vi "GUI_Final.vi"() -> ()   [LabVIEW 2013]
uses:
  <vilib>/Instr/_visa.llb/VISA Configure Serial Port (Instr).vi
panel:
  out "Angle":u8[](array[numeric])
  out "Left":bool
  out "Right":bool
  out "read buffer":string
  in  "Stop":bool
  in  "Angle":string
  out "Error":errorcluster
  out "Arduino Data":string
  in  "Mode":bool
  in  "Baud Rate 2":u32=9600
  in  "Port 2":refnum<visa-resource-name>
  in  "Baud Rate":u32=9600
  in  "Port":refnum<visa-resource-name>
  out "Response 2":string
  in  "Command":string
  out "error out":errorcluster
  out "Numeric 12":i32
  in  "angle":i32
  in  "OK":bool
  in  "Commands":string(combo)
  out "error out 2":errorcluster
  in  "MODE":bool
  # "Arduino Interface"
  # "Encoder Interface"
  # "Text Mode"
  # "Button Mode"
  # "Select : ON : Text Mode , \n              OFF : ButtonMode"
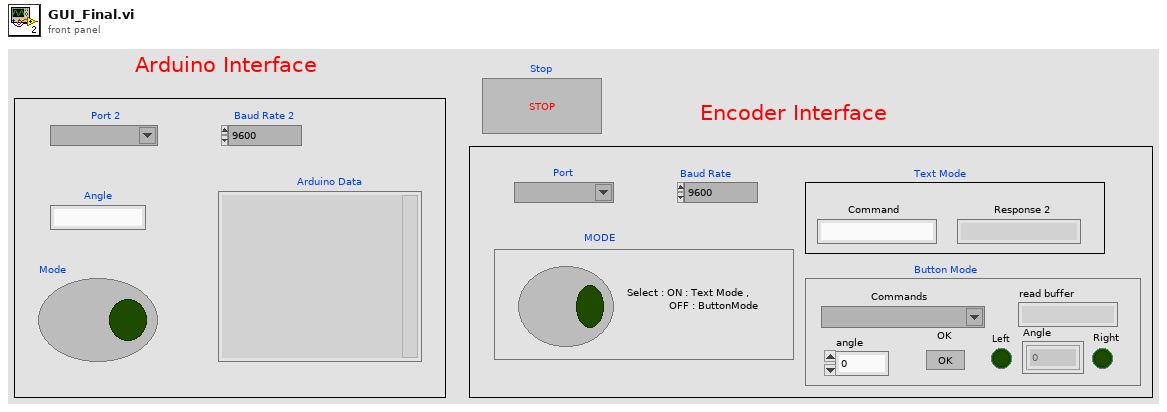
[diagram p1: front panel]
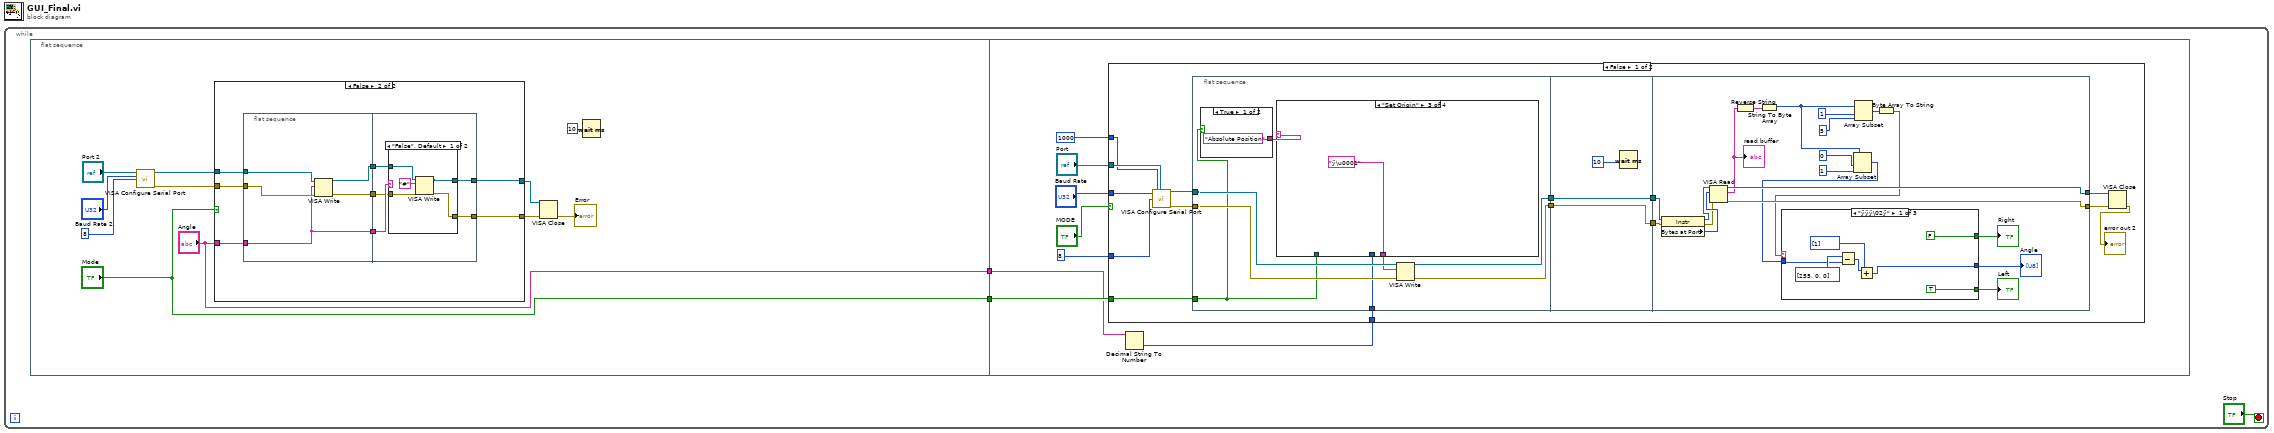
[diagram p0: block diagram]
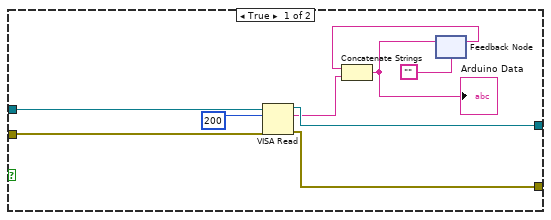
[diagram p2: hidden frame]
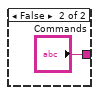
[diagram p4: hidden frame]
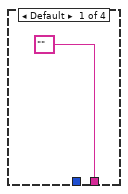
[diagram p5: hidden frame]
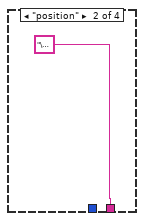
[diagram p6: hidden frame]
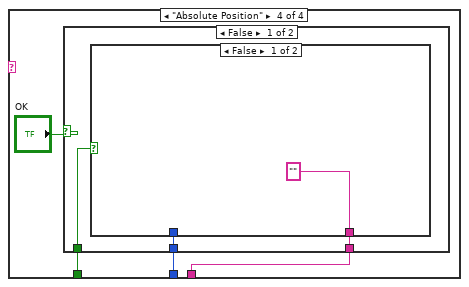
[diagram p7: hidden frame]
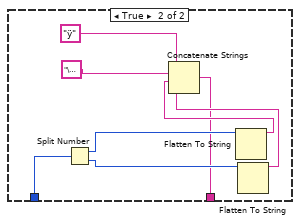
[diagram p8: hidden frame]
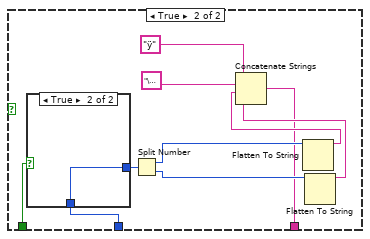
[diagram p9: hidden frame]
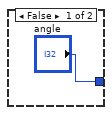
[diagram p10: hidden frame]
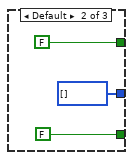
[diagram p11: hidden frame]
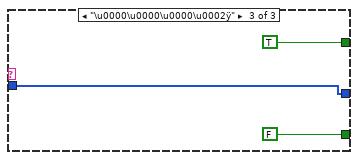
[diagram p12: hidden frame]
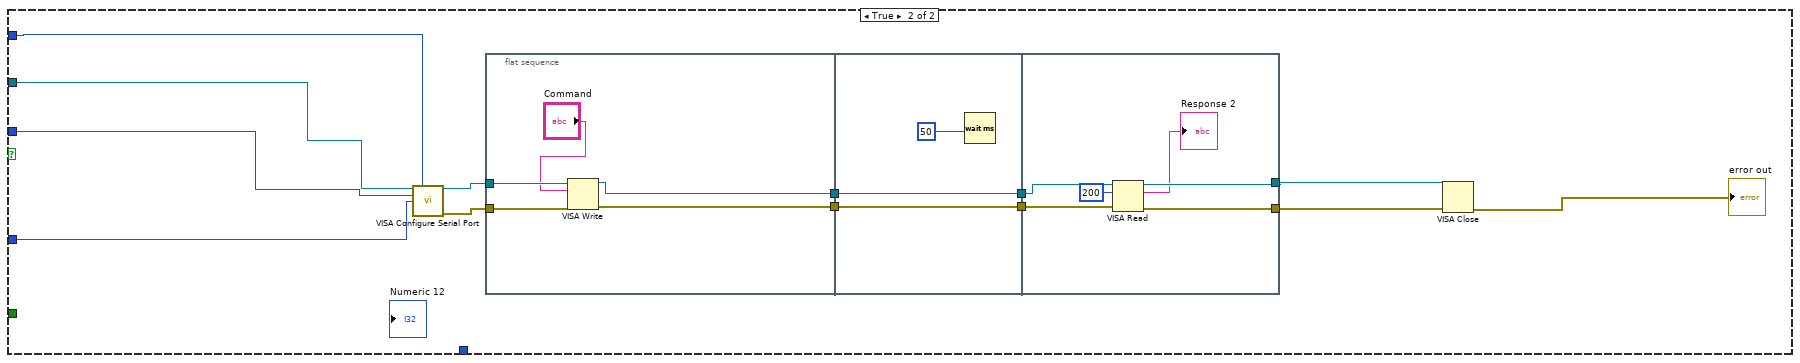
[diagram p13: hidden frame]
diagram:
  n1 = while {
    stop <- "Stop" stop-if-true
    n2 = flat-sequence {
      tunnel: ["Mode"] -> w3
      tunnel: ["Angle"] -> w2
      tunnel: w3 -> [w52]
      tunnel: w2 -> [w51]
      frame #0 {
        n3 = call-poly "VISA Configure Serial Port"("VISA resource name"="Port 2", "baud rate (9600)"="Baud Rate 2", "data bits (8)"=u16 8) -> ("VISA resource name out"=w6:refnum<visa-resource-name>, "error out"=w7:errorcluster)  [unwired: 11 in]
        n4 = case shown="False" "Mode" {
          tunnel: w6 -> [w21 w31]
          tunnel: [w22 w25] -> w13
          tunnel: [w23 w26] -> w14
          tunnel: w7 -> [w20 w30]
          tunnel: "Angle" -> [_ w24]
          frame True {
            n5 = VISA Read(VISA resource name=w21, byte count=u32 200, error in (no error)=w20) -> (VISA resource name out=w23:refnum<visa-resource-name>, read buffer=w18:string, error out=w22:errorcluster)  [unwired: 1 out]
            n6 = feedback #1("") -> (w17:string)
            n7 = Concatenate Strings(w17, w18) -> (w16:string)
            "Arduino Data" <- w16
            n8 = feedback-in #1(w16) -> ()
          }
          frame False {
            n9 = flat-sequence {
              tunnel: w31 -> [w36]
              tunnel: w30 -> [w35]
              tunnel: [w32] -> w29
              tunnel: [w34] -> w28
              tunnel: [w33] -> w27
              tunnel: w24 -> [w32]
              tunnel: w29 -> [w41]
              tunnel: w28 -> [w40]
              tunnel: w27 -> [w39]
              tunnel: [w38] -> w26
              tunnel: [w37] -> w25
              frame #0 {
                n10 = VISA Write(VISA resource name=w36, write buffer=w32, error in (no error)=w35) -> (VISA resource name out=w34:refnum<visa-resource-name>, error out=w33:errorcluster)  [unwired: 1 out]
              }
              frame #1 {
                n11 = case shown="\"False\", Default" w41 {
                  tunnel: w40 -> [w45 w48]
                  tunnel: w39 -> [w44 w47]
                  tunnel: [w43 w48] -> w38
                  tunnel: [w42 w47] -> w37
                  frame "False", Default {
                    n12 = VISA Write(VISA resource name=w45, write buffer="#", error in (no error)=w44) -> (VISA resource name out=w43:refnum<visa-resource-name>, error out=w42:errorcluster)  [unwired: 1 out]
                  }
                  frame "" {
                  }
                }
              }
            }
          }
        }
        n13 = VISA Close(VISA resource name=w14, error in (no error)=w13) -> (error out=→"Error":errorcluster)
        n14 = Wait (ms)(milliseconds to wait=u32 10) -> ()  [unwired: 1 out]
      }
      frame #1 {
        n15 = Decimal String To Number(string=w51) -> (number=w49:i32)  [unwired: 2 in, 1 out]
        n16 = case shown="False" "MODE" {
          tunnel: u32 1000 ("timeout (10sec)") -> [w57 w152]
          tunnel: "Port" -> [w65 w151]
          tunnel: "Baud Rate" -> [w64 w150]
          tunnel: u16 8 ("data bits (8)") -> [w59 w149]
          tunnel: w52 -> [w63 _]
          tunnel: w49 -> [w58 _]
          frame False {
            n17 = call-poly "VISA Configure Serial Port"("VISA resource name"=w65, "timeout (10sec)"=w57, "baud rate (9600)"=w64, "data bits (8)"=w59) -> ("VISA resource name out"=w69:refnum<visa-resource-name>, "error out"=w68:errorcluster)  [unwired: 10 in]
            n18 = flat-sequence {
              tunnel: [w78] -> w71
              tunnel: w69 -> [w77]
              tunnel: w68 -> [w76]
              tunnel: [w79] -> w67
              tunnel: w63 -> [w73]
              tunnel: w58 -> [w72]
              tunnel: [w114] -> w70
              tunnel: w71 -> [w113]
              tunnel: w67 -> [w114]
              tunnel: [w113] -> w66
              tunnel: w70 -> [w121]
              tunnel: [w135] -> w61
              tunnel: [w134] -> w62
              tunnel: w66 -> [w132]
              frame #0 {
                n19 = case shown="True" w73 {
                  tunnel: ["Absolute Position" ("Commands") "Commands"] -> w75
                  frame True {
                  }
                  frame False {
                  }
                }
                n20 = case shown="\"Set Origin\"" w75 {
                  tunnel: ["" "\u001f" "ÿ\u0001" w85] -> w74
                  tunnel: w73 -> [_ _ _ w87]
                  tunnel: w72 -> [_ _ _ w86]
                  frame Default {
                  }
                  frame "position" {
                  }
                  frame "Set Origin" {
                  }
                  frame "Absolute Position" {
                    n21 = case shown="False" "OK" {
                      tunnel: w87 -> [w91 w103]
                      tunnel: w86 -> [w90 w101]
                      tunnel: [w89 w102] -> w85
                      frame False {
                        n22 = case shown="False" w91 {
                          tunnel: w90 -> [_ w94]
                          tunnel: ["" w93] -> w89
                          frame False {
                          }
                          frame True {
                            n23 = Split Number(x=w94) -> (hi(x)=w96:u16, lo(x)=w95:u16)
                            n24 = Flatten To String(anything=w96) -> (data string=w98:string)  [unwired: 3 in, 2 out]
                            n25 = Flatten To String(anything=w95) -> (data string=w97:string)  [unwired: 3 in, 2 out]
                            n26 = Concatenate Strings("ÿ" ("string"), "\u0002" ("string"), w98, w97) -> (w93:string)
                          }
                        }
                      }
                      frame True {
                        n27 = case shown="True" w103 {
                          tunnel: w101 -> [_ w112]
                          tunnel: ["angle" w112] -> w104
                          frame False {
                          }
                          frame True {
                          }
                        }
                        n28 = Split Number(x=w104) -> (hi(x)=w106:u16, lo(x)=w105:u16)
                        n29 = Flatten To String(anything=w106) -> (data string=w108:string)  [unwired: 3 in, 2 out]
                        n30 = Flatten To String(anything=w105) -> (data string=w107:string)  [unwired: 3 in, 2 out]
                        n31 = Concatenate Strings("ÿ" ("string"), "\u0002" ("string"), w108, w107) -> (w102:string)
                      }
                    }
                  }
                }
                n32 = VISA Write(VISA resource name=w77, write buffer=w74, error in (no error)=w76) -> (VISA resource name out=w79:refnum<visa-resource-name>, error out=w78:errorcluster)  [unwired: 1 out]
              }
              frame #1 {
                n33 = Wait (ms)(milliseconds to wait=u32 10) -> ()  [unwired: 1 out]
              }
              frame #2 {
                n34 = property class="Instr"(reference=w121, error in=w132) -> (reference out=w120:refnum<visa-resource-name>, error out=w131:errorcluster, "Bytes at Port"=w133:u32)
                n35 = VISA Read(VISA resource name=w120, byte count=w133, error in (no error)=w131) -> (VISA resource name out=w134:refnum<visa-resource-name>, read buffer=w127:string, error out=w135:errorcluster)  [unwired: 1 out]
                "read buffer" <- w127
                n36 = Reverse String(1:w127) -> (0:w119:string)
                n37 = String To Byte Array(string=w119) -> (unsigned byte array=w130:u8[])
                n38 = Array Subset(array=w130, index=0, length=1) -> (w122:u8[])
                n39 = Array Subset(array=w130, index=1, length=5) -> (w123:u8[])
                n40 = Byte Array To String(unsigned byte array=w123) -> (string=w128:string)
                n41 = case shown="\"ÿÿÿ\\02ÿ\"" w128 {
                  tunnel: w122 -> [w139 _ w148]
                  tunnel: [w138 u8[] [] w148] -> w124
                  tunnel: [TRUE ("Boolean") FALSE ("Boolean") FALSE ("Boolean")] -> w126
                  tunnel: [FALSE ("Boolean") FALSE ("Boolean") TRUE ("Boolean")] -> w125
                  frame "ÿÿÿ\u0002ÿ" {
                    n42 = Subtract(x=u8[] [255, 0, 0] ("y"), y=w139) -> (x-y=w142:u8[])
                    n43 = Add(x=w142, y=u8[] [1]) -> (x+y=w138:u8[])
                  }
                  frame Default {
                  }
                  frame "\u0000\u0000\u0000\u0002ÿ" {
                  }
                }
                "Left" <- w126
                "Right" <- w125
                "Angle" <- w124
              }
            }
            n44 = VISA Close(VISA resource name=w62, error in (no error)=w61) -> (error out=→"error out 2":errorcluster)
          }
          frame True {
            n45 = call-poly "VISA Configure Serial Port"("VISA resource name"=w151, "timeout (10sec)"=w152, "baud rate (9600)"=w150, "data bits (8)"=w149) -> ("VISA resource name out"=w157:refnum<visa-resource-name>, "error out"=w156:errorcluster)  [unwired: 10 in]
            n46 = flat-sequence {
              tunnel: w157 -> [w164]
              tunnel: w156 -> [w166]
              tunnel: [w163] -> w161
              tunnel: [w165] -> w160
              tunnel: [w168] -> w159
              tunnel: w161 -> [w168]
              tunnel: [w167] -> w158
              tunnel: w160 -> [w167]
              tunnel: w159 -> [w175]
              tunnel: w158 -> [w174]
              tunnel: [w173] -> w154
              tunnel: [w172] -> w155
              frame #0 {
                n47 = VISA Write(VISA resource name=w164, write buffer="Command", error in (no error)=w166) -> (VISA resource name out=w163:refnum<visa-resource-name>, error out=w165:errorcluster)  [unwired: 1 out]
              }
              frame #1 {
                n48 = Wait (ms)(milliseconds to wait=u32 50) -> ()  [unwired: 1 out]
              }
              frame #2 {
                n49 = VISA Read(VISA resource name=w175, byte count=u32 200, error in (no error)=w174) -> (VISA resource name out=w172:refnum<visa-resource-name>, read buffer=→"Response 2":string, error out=w173:errorcluster)  [unwired: 1 out]
              }
            }
            n50 = VISA Close(VISA resource name=w155, error in (no error)=w154) -> (error out=→"error out":errorcluster)
          }
        }
      }
    }
  }
